vi "客户机.vi"() -> ()   [LabVIEW 2017]
panel:
  in  "停止":bool
  out "波形图":dbl[](graph)
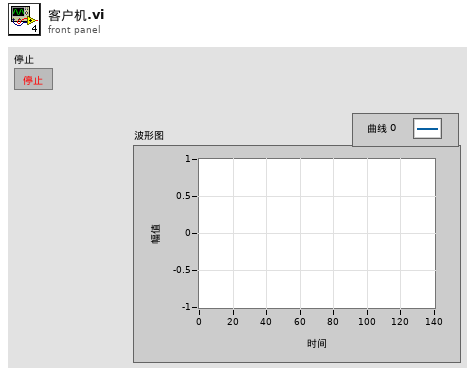
[diagram p1: front panel]
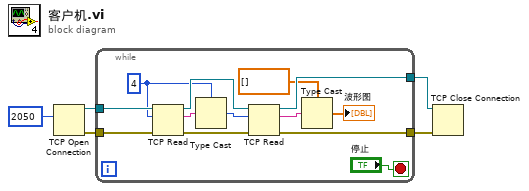
[diagram p0: block diagram]
diagram:
  n1 = TCP Open Connection(remote port or service name=u16 2050 ("远程端口或服务名称")) -> (connection ID=w5:refnum<k5>, error out=w4:errorcluster)  [unwired: 4 in]
  n2 = while {
    tunnel: w5 -> [w18]
    tunnel: w4 -> [w17]
    tunnel: [w14] -> w2
    tunnel: [w13] -> w1
    stop <- "停止" stop-if-true
    w11 = 4
    n3 = TCP Read(connection ID=w18, bytes to read=w11, error in (no error)=w17) -> (connection ID out=w16:refnum<k5>, data out=w12:string, error out=w15:errorcluster)  [unwired: 2 in]
    n4 = Type Cast(type=w11, x=w12) -> (*(type *) &x=w10:i32)
    n5 = TCP Read(connection ID=w16, bytes to read=w10, error in (no error)=w15) -> (connection ID out=w14:refnum<k5>, data out=w8:string, error out=w13:errorcluster)  [unwired: 2 in]
    n6 = Type Cast(type=dbl[] [], x=w8) -> (*(type *) &x=→"波形图":dbl[])
  }
  n7 = TCP Close Connection(connection ID=w2, error in (no error)=w1) -> ()  [unwired: 1 in, 2 out]
